vi "CTRE_Phoenix_CANdle_FactoryDefault.vi"(6 "timeoutMs":i32, 8 "error in":errorcluster, 11 "CTRE_CANdle_DeviceRef":T1) -> (0 "error out":errorcluster, 3 "CTRE_CANdle_DeviceRef":T1)   [LabVIEW 2020]
doc: "Reset all configurations to factory default value"
uses:
  <vilib>/Rock Robotics/WPI/ThirdParty/Phoenix-LabVIEW/CANdle/Controls/CTRE_Phoenix_CANdle_DeviceRef.ctl
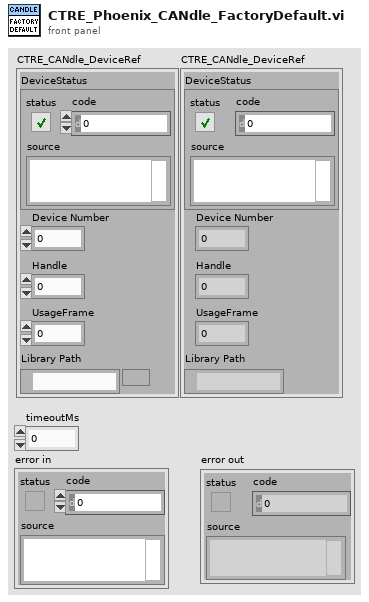
[diagram p1: front panel]
types:
  T1 = typedef "CTRE_Phoenix_CANdle_DeviceRef.ctl" = cluster{"DeviceStatus":errorcluster, "Device Number":u8, "Handle":u64, "UsageFrame":u32, "Library Path":path}
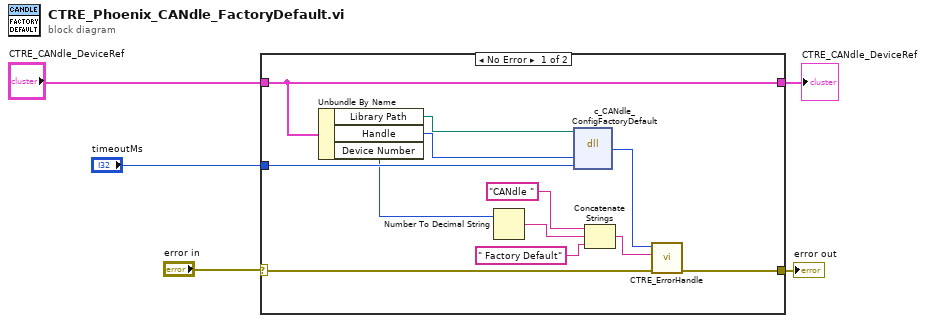
[diagram p0: block diagram]
diagram:
  n1 = case shown="No Error" "error in" {
    selector: "error in" -> [w15 w19]
    tunnel: "CTRE_CANdle_DeviceRef" -> [w13 w18]
    tunnel: "timeoutMs" -> [w17 _]
    tunnel: [w14 w19] -> w3
    tunnel: [w13 w18] -> w1
    frame No Error {
      n2 = Unbundle By Name(w13) -> ("Library Path"=w12:path, "Handle"=w11:u64, "Device Number"=w6:u8)
      n3 = Number To Decimal String(number=w6) -> (decimal integer string=w10:string)  [unwired: 1 in]
      n4 = dll-call lib="?" fn="c_CANdle_ConfigFactoryDefault"(path in=w12, "handle"=w11, "timeoutMs"=w17) -> ("ErrorCode"=w16:i32)  [unwired: 4 in, 2 out]
      n5 = Concatenate Strings("CANdle " ("string"), w10, " Factory Default" ("string")) -> (w7:string)
      n6 = call <vilib>:"CTRE_ErrorHandle.vi"("error in"=w15, "origin"=w7, "code"=w16) -> ("error out"=w14:errorcluster)  [unwired: 8 in]
    }
    frame Error {
    }
  }
  "error out" <- w3
  "CTRE_CANdle_DeviceRef" <- w1
